vi "Release Sum Handles.vi"(8 "error in (no error)":errorcluster, 9 "Handles":u32[](array[numeric]), 11 "TwinCAT ADS in":refnum<class "TwinCAT ADS.lvclass">) -> (0 "error out":errorcluster, 3 "TwinCAT ADS out":refnum<class "TwinCAT ADS.lvclass">)   [LabVIEW 2018, in "TwinCAT ADS.lvclass"]
uses:
  TwinCAT ADS.lvclass
  TwinCAT.Ads
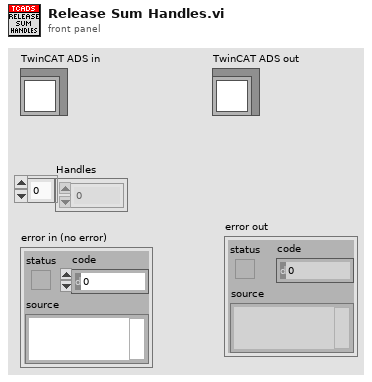
[diagram p1: front panel]
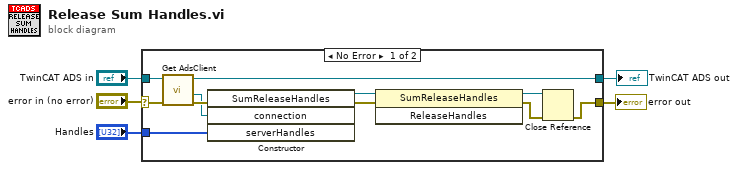
[diagram p0: block diagram]
diagram:
  n1 = case shown="No Error" "error in (no error)" {
    selector: "error in (no error)" -> [w15 w18]
    tunnel: [w14 w18] -> w4
    tunnel: [w10 w17] -> w2
    tunnel: "TwinCAT ADS in" -> [w16 w17]
    tunnel: "Handles" -> [w6 _]
    frame No Error {
      n2 = call-dynamic "Get AdsClient.vi"("error in (no error)"=w15, "TwinCAT ADS in"=w16) -> ("error out"=w12:errorcluster, ".NET TcAdsClient refnum"=w11:refnum<k24>, "TwinCAT ADS out"=w10:refnum<class "TwinCAT ADS.lvclass">)  [unwired: 7 in]
      n3 = constructor class="SumReleaseHandles"(error in=w12, "connection"=w11, "serverHandles"=w6) -> (reference out=w7:refnum<k24>, error out=w13:errorcluster)  [unwired: 2 in, 3 out]
      n4 = invoke class="SumReleaseHandles" method="ReleaseHandles"(reference=w7, error in=w13) -> (reference out=w8:refnum<k24>, error out=w9:errorcluster)  [unwired: 1 in, 1 out]
      n5 = Close Reference(reference=w8, error in (no error)=w9) -> (error out=w14:errorcluster)
    }
    frame Error {
    }
  }
  "error out" <- w4
  "TwinCAT ADS out" <- w2
